vi "dfd_DFXP Use Double (vector).vi"(9 "Value in 2":T1, 10 "Value in":T1) -> (1 "Result wl":i16, 2 "Use 64?":bool, 3 "Use double?":bool)   [LabVIEW 2017, in "NI_DigFilter_FXP.lvlib"]
uses:
  <vilib>/addons/Digital Filter Design/NI_DigFilter_FXP.lvlib
  <vilib>/addons/Digital Filter Design/_Objects.llb/dfd_DFXP Data Type (vector).ctl
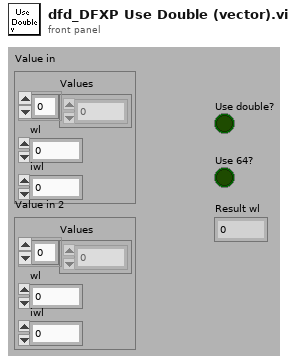
[diagram p1: front panel]
types:
  T1 = typedef "dfd_DFXP Data Type (vector).ctl" = cluster{"Values":i64[], "wl":i16, "iwl":i16}
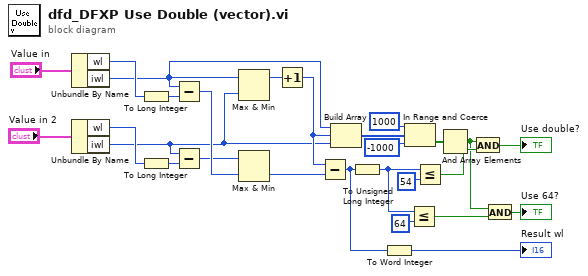
[diagram p0: block diagram]
diagram:
  n1 = Unbundle By Name("Value in") -> ("wl"=w19:i16, "iwl"=w16:i16)
  n2 = Unbundle By Name("Value in 2") -> ("wl"=w18:i16, "iwl"=w14:i16)
  n3 = To Long Integer(number=w19) -> (32bit integer=w25:i32)
  n4 = To Long Integer(number=w18) -> (32bit integer=w24:i32)
  n5 = Subtract(x=w16, y=w25) -> (x-y=w23:i32)
  n6 = Subtract(x=w14, y=w24) -> (x-y=w22:i32)
  n7 = Max & Min(x=w16, y=w14) -> (max(x,y)=w21:i16)  [unwired: 1 out]
  n8 = Max & Min(x=w22, y=w23) -> (min(x,y)=w20:i32)  [unwired: 1 out]
  n9 = Increment(x=w21) -> (x+1=w15:i16)
  n10 = Subtract(x=w15, y=w20) -> (x-y=w3:i32)
  n11 = Build Array(w16, w15, w14) -> (w11:i16[])
  n12 = To Unsigned Long Integer(number=w3) -> (unsigned 32bit integer=w2:u32)
  n13 = To Word Integer(number=w3) -> (16bit integer=→"Result wl":i16)
  n14 = In Range and Coerce(upper limit=1000 ("y"), x=w11, lower limit=-1000 ("y")) -> (In Range?=w9:bool[])  [unwired: 1 out]
  n15 = Less Or Equal?(x=w2, y=u32 64) -> (x <= y?=w6:bool)
  n16 = Less Or Equal?(x=w2, y=u32 54) -> (x <= y?=w10:bool)
  n17 = And Array Elements(Boolean array=w9) -> (logical AND=w1:bool)
  n18 = And(x=w1, y=w10) -> (x .and. y?=→"Use double?":bool)
  n19 = And(x=w1, y=w6) -> (x .and. y?=→"Use 64?":bool)
